vi "getPoints.vi"(8 "error in (no error)":errorcluster, 11 "Polygon in":refnum<class "Polygon.lvclass">) -> (0 "error out":errorcluster, 2 "Points":cluster{"X":dbl, "Y":dbl}[](array[cluster]), 3 "Polygon out":refnum<class "Polygon.lvclass">)   [LabVIEW 2014, in "Polygon.lvclass"]
uses:
  <userlib>/AdvancedDataStructures/ClassBased/Applications/Occupancy/Polygon/Polygon.lvclass
  <userlib>/AdvancedDataStructures/ClassBased/Applications/Occupancy/Polygon/Polygon.lvclass/Polygon.ctl
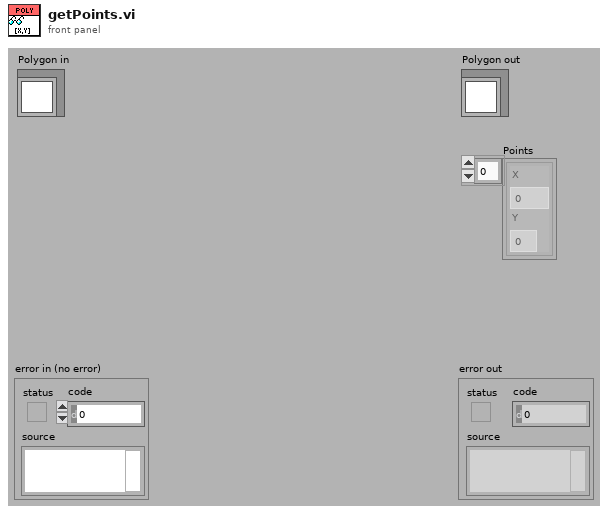
[diagram p1: front panel]
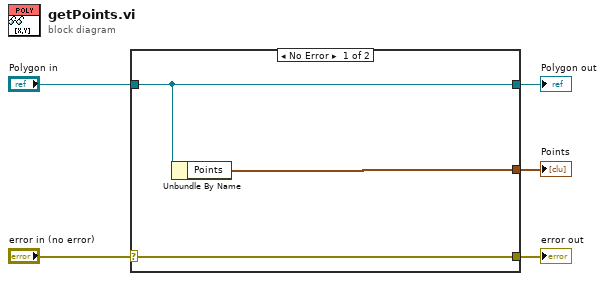
[diagram p0: block diagram]
diagram:
  n1 = case shown="No Error" "error in (no error)" {
    selector: "error in (no error)" -> [w8 w9]
    tunnel: [w8 w9] -> w4
    tunnel: [w7 w10] -> w2
    tunnel: "Polygon in" -> [w7 w10]
    tunnel: [w6 _] -> w1
    frame No Error {
      n2 = Unbundle By Name(w7) -> ("Points"=w6:cluster{"X":dbl, "Y":dbl}[])
    }
    frame Error {
    }
  }
  "error out" <- w4
  "Polygon out" <- w2
  "Points" <- w1
